vi "Init.vi"(11 "Online?":bool) -> (0 "Fehler out":T1, 1 "SPS-Event":refnum<user-event>, 2 "Version":string, 3 "Cluster out":T2={"Initialisierung"={"Online?"=FALSE, "Grundpfad"=path "", "Kamera Oben"="", "IP-Adresse Flüssiglinse"="", "Flüssiglinse"=refnum, "Kamera Unten"="", "IP-Adresse SPS"="", "SPS-Verbindung"={"TCP Connection Ref"=refnum, "IP address"="", "timeout ms"=5000, "Connected?"=FALSE, "PLC Type"=enum."S7 1200", "Rack S7 400"=0, "Slot S7 400"=0, "PDU Size"=0, "connection semaphore"=refnum}, "IP-Adresse Lichtgitter"="", "Lichtgitter"=refnum, "Skalierungsfaktor"=0.0, "Bilder Oben"=[], "Bild Unten"=refnum, "Bild Ausschnitt Unten"=refnum}, "Einstellungen"={"Gesamtablauf gestartet"=FALSE, "i. O. Bilder speichern"=FALSE, "Bildspeicherung Offline"=FALSE, "Ausgewähltes Offline-Datum"="", "Ausgewähltes Offline-Teil"="", "Speicherpfad Bilder"=path ""}, "Artikeldaten"={"Artikelnummer"="", "Fertigungsauftrag"="", "Muster ISO"=refnum, "Belichtungszeit Referenzmarken"=0.0, "Fokus Referenzmarken"=0.0, "Belichtungszeit ISO"=0.0, "Fokus ISO"=0.0, "Belichtungszeit Unten"=0.0, "Kontaktanzahl"=0, "Aktueller Kontakt"=0, "Kontaktposition"={"x"=0.0, "y"=0.0}, "Winkel ISO"=0.0, "ISO-Muster nicht vorhanden"=FALSE}, "Werte Kamera Oben"={"Koordinatensystem"={"Punkt x-Achse"={"X"=0.0, "Y"=0.0}, "Ursprung"={"X"=0.0, "Y"=0.0}, "Punkt y-Achse"={"X"=0.0, "Y"=0.0}}, "Position Kontakt"={"x"=0.0, "y"=0.0}, "Winkel Kontakt"=0.0}, "Werte Kamera Unten"={"Prüfung Unten n. i. O."=FALSE}, "Werte Lichtgitter"={"Messwerte Referenzmarken"=[], "Mittelpunkt Referenzmarken"={"x"=0.0, "y"=0.0}, "Messwerte Kontakt"=[], "Offset"={"x"=0.0, "y"=0.0}}, "Rückmeldungen"={"Koordinaten ermittelt"=FALSE, "Vermessung Lichtgitter fertig"=FALSE, "Nachkontrolle Kamera Unten fertig"=FALSE}, "Fehler"={"Referenzen nicht gefunden"=FALSE, "Kontakt nicht gefunden"=FALSE, "Referenzen nicht in Lichtgitter"=FALSE, "Kontakt zu groß"=FALSE, "Kontakt zu klein"=FALSE}, "Statistik"={"Statistiken"=[]}, "Timer"={"Timer Start Position"=0, "Timer Start Lichtgitter"=0, "Timer Start Kamera Unten"=0}})   [LabVIEW 2024]
doc: "Verbindet alle Geräte und initialisiert Grundvariablen"
uses:
  Cluster.ctl
  Kontaktmontagemodul.exe/1abvi3w/vi.lib/userDefined/High Color/IMAQdx.ctl
  Kontaktmontagemodul.exe/1abvi3w/vi.lib/DATA AHEAD/SP7/typedefs/S7 Connection.ctl
  Kontaktmontagemodul.exe/1abvi3w/vi.lib/DATA AHEAD/SP7/typedefs/PLC Type.ctl
  Kontaktmontagemodul.exe/1abvi3w/vi.lib/vision/Image Controls.llb/IMAQ Image.ctl
  Koordinatensystem.ctl
  Statistik.ctl
  Cluster_Fehler_Initialisierung.ctl
  Zustand.ctl
  Globale Variablen.vi
  Kontaktmontagemodul.exe/1abvi3w/vi.lib/DATA AHEAD/SP7/SP7.lvlib
  Kontaktmontagemodul.exe/1abvi3w/vi.lib/vision/driver/NI_Vision_Acquisition_Software.lvlib
  Kontaktmontagemodul.exe/1abvi3w/vi.lib/Utility/config.llb/NI_LVConfig.lvlib
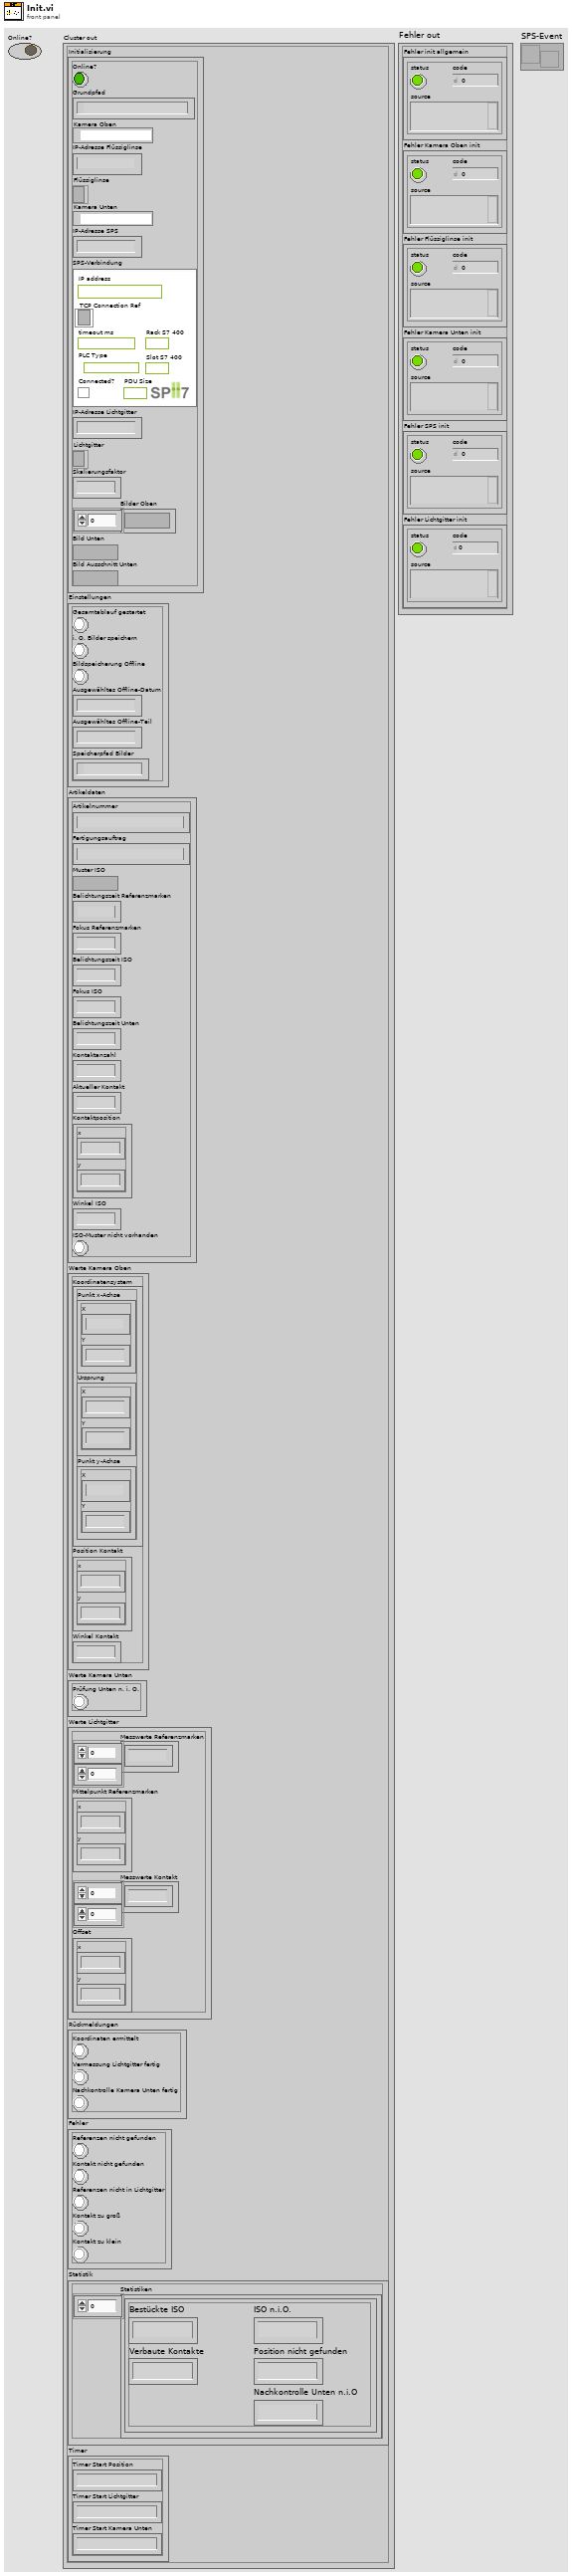
[diagram p1: front panel]
types:
  T1 = typedef "Cluster_Fehler_Initialisierung.ctl" = cluster{"Fehler init allgemein":errorcluster, "Fehler Kamera Oben init":errorcluster, "Fehler Flüssiglinse init":errorcluster, "Fehler Kamera Unten init":errorcluster, "Fehler SPS init":errorcluster, "Fehler Lichtgitter init":errorcluster}
  T2 = typedef "Cluster.ctl" = cluster{"Initialisierung":cluster{"Online?":bool, "Grundpfad":path, "Kamera Oben":T3, "IP-Adresse Flüssiglinse":string, "Flüssiglinse":refnum<k5>, "Kamera Unten":T3, "IP-Adresse SPS":string, "SPS-Verbindung":T4, "IP-Adresse Lichtgitter":string, "Lichtgitter":refnum<k5>, "Skalierungsfaktor":dbl, "Bilder Oben":T7[], "Bild Unten":T7, "Bild Ausschnitt Unten":T7}, "Einstellungen":cluster{"Gesamtablauf gestartet":bool, "i. O. Bilder speichern":bool, "Bildspeicherung Offline":bool, "Ausgewähltes Offline-Datum":string, "Ausgewähltes Offline-Teil":string, "Speicherpfad Bilder":path}, "Artikeldaten":cluster{"Artikelnummer":string, "Fertigungsauftrag":string, "Muster ISO":T7, "Belichtungszeit Referenzmarken":dbl, "Fokus Referenzmarken":dbl, "Belichtungszeit ISO":dbl, "Fokus ISO":dbl, "Belichtungszeit Unten":dbl, "Kontaktanzahl":u32, "Aktueller Kontakt":i16, "Kontaktposition":cluster{"x":sgl, "y":sgl}, "Winkel ISO":sgl, "ISO-Muster nicht vorhanden":bool}, "Werte Kamera Oben":cluster{"Koordinatensystem":T8, "Position Kontakt":cluster{"x":dbl, "y":dbl}, "Winkel Kontakt":dbl}, "Werte Kamera Unten":cluster{"Prüfung Unten n. i. O.":bool}, "Werte Lichtgitter":cluster{"Messwerte Referenzmarken":dbl[][], "Mittelpunkt Referenzmarken":cluster{"x":dbl, "y":dbl}, "Messwerte Kontakt":dbl[][], "Offset":cluster{"x":dbl, "y":dbl}}, "Rückmeldungen":cluster{"Koordinaten ermittelt":bool, "Vermessung Lichtgitter fertig":bool, "Nachkontrolle Kamera Unten fertig":bool}, "Fehler":cluster{"Referenzen nicht gefunden":bool, "Kontakt nicht gefunden":bool, "Referenzen nicht in Lichtgitter":bool, "Kontakt zu groß":bool, "Kontakt zu klein":bool}, "Statistik":cluster{"Statistiken":T9[]}, "Timer":cluster{"Timer Start Position":u32, "Timer Start Lichtgitter":u32, "Timer Start Kamera Unten":u32}}
  T3 = typedef "IMAQdx.ctl" = refnum<k21>
  T4 = typedef "SP7.lvlib/S7 Connection.ctl" = cluster{"TCP Connection Ref":refnum<k5>, "IP address":string, "timeout ms":i32, "Connected?":bool, "PLC Type":T5, "Rack S7 400":u8, "Slot S7 400":u8, "PDU Size":u16, "connection semaphore":T6}
  T5 = typedef "SP7.lvlib/PLC Type.ctl" = enum16{"S7 200", "S7 300/400", "S7 1200", "S7 1500", "LOGO!8"}
  T6 = typedef "Semaphore RefNum" = refnum<k1>
  T7 = typedef "IMAQ Image.ctl" = refnum<image>
  T8 = typedef "Koordinatensystem.ctl" = cluster{"Punkt x-Achse":cluster{"X":sgl, "Y":sgl}, "Ursprung":cluster{"X":sgl, "Y":sgl}, "Punkt y-Achse":cluster{"X":sgl, "Y":sgl}}
  T9 = typedef "Statistik.ctl" = cluster{"Bestückte ISO":u32, "Verbaute Kontakte":u32, "ISO n.i.O.":u32, "Nachkontrolle Unten n.i.O":u32, "Position nicht gefunden":u32}
  T10 = typedef "Zustand.ctl" = enum16{"Warten auf Event", "Artikeldaten laden", "Init Prüfung Oben", "Bildaufnahme Oben", "Auswertung Oben", "Bilder Oben speichern", "Init Vermessung Lichtgitter", "Messwertaufnahme Lichtgitter", "Auswertung Lichtgitter", "Init Prüfung Unten", "Bildaufnahme Unten", "Auswertung Unten", "Bild Unten speichern", "Update Statistik", "Fehler quittieren"}
  T11 = typedef "NI_LVConfig.lvlib/Config Data RefNum.ctl" = refnum<k1>
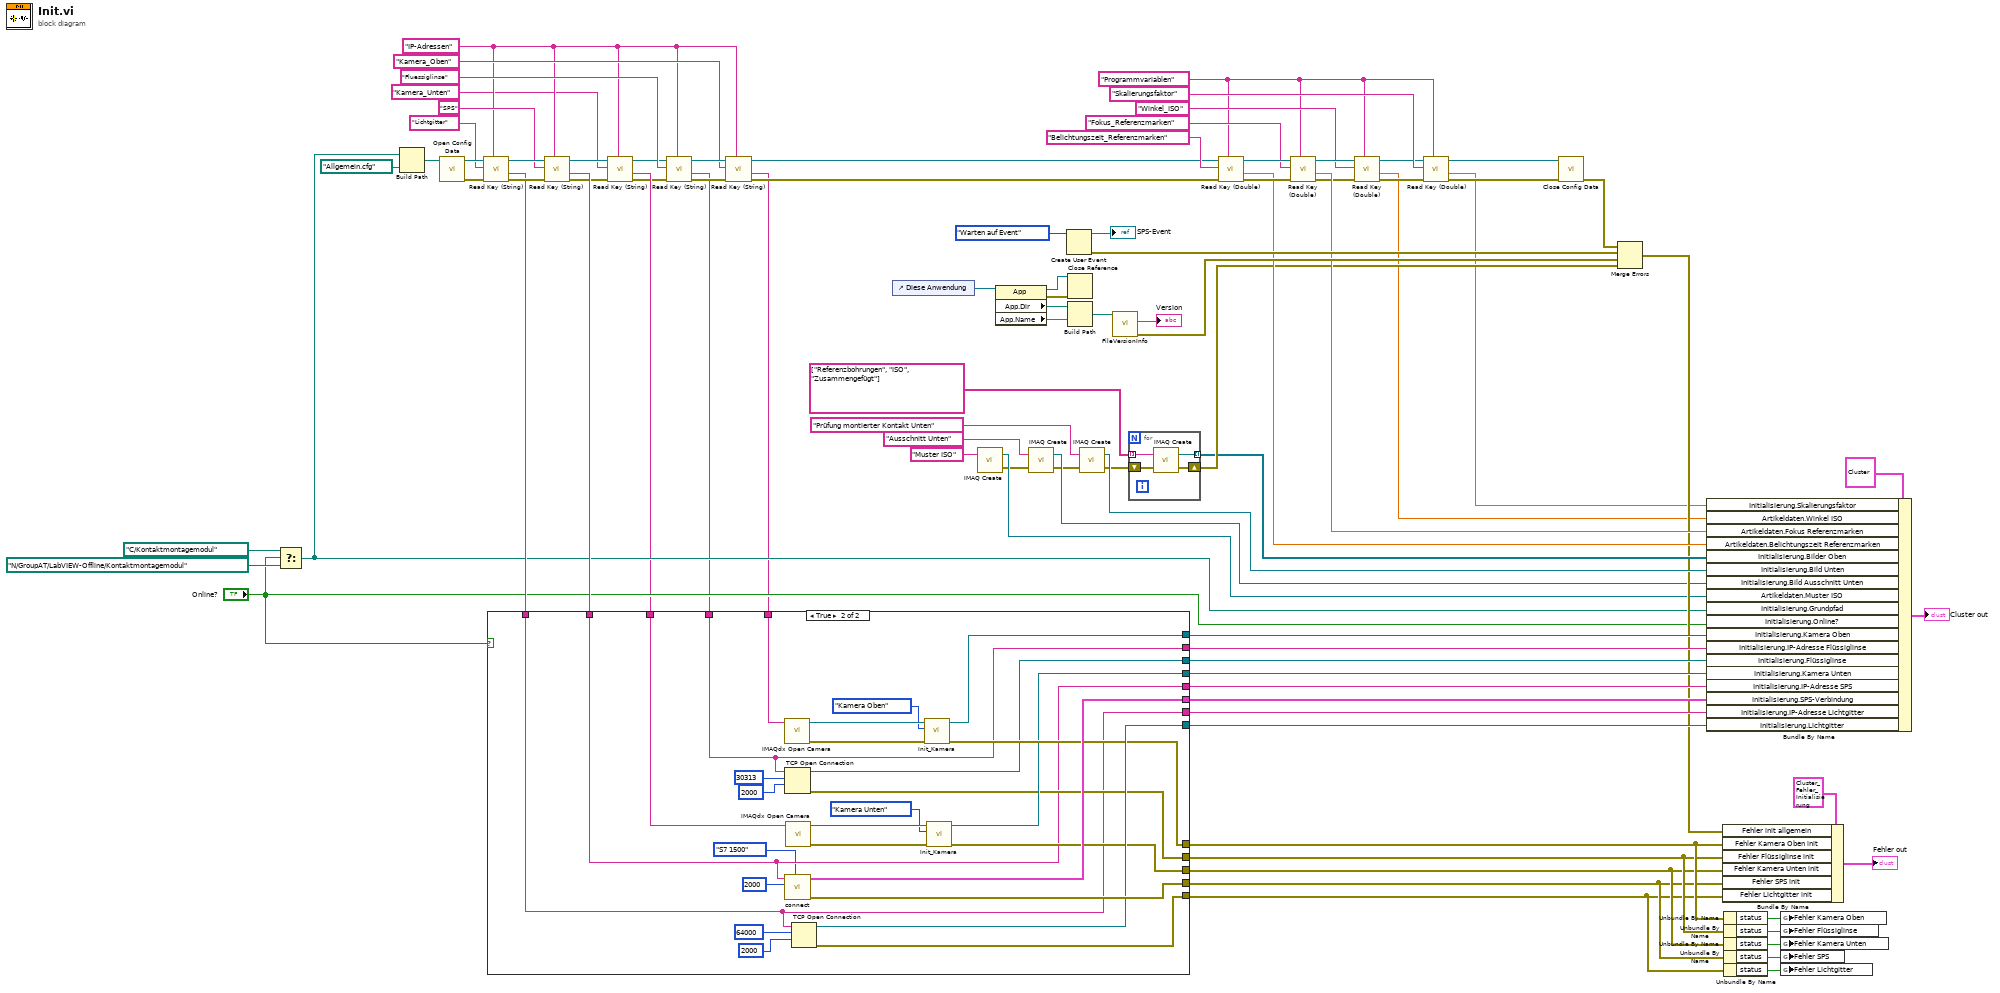
[diagram p0: block diagram]
diagram:
  w21 = "IP-Adressen" ("section")
  w3 = "Programmvariablen" ("section")
  n1 = Select(t=path "C:/Kontaktmontagemodul", s="Online?", f=path "N:/GroupAT/LabVIEW-Offline/Kontaktmontagemodul") -> (s? t:f=w33:path)
  n2 = Build Path(base path=w33, name or relative path=path "Allgemein.cfg") -> (appended path=w67:path)
  n3 = call "Open Config Data.vi"("configuration file path"=w67) -> ("error out"=w52:errorcluster, "refnum"=w53:T11)  [unwired: 8 in, 1 out]
  n4 = call "Read Key (String).vi"("section"=w21, "error in (no error)"=w52, "key"="Lichtgitter", "refnum"=w53) -> ("error out"=w50:errorcluster, "value"=w45:string, "refnum out"=w51:T11)  [unwired: 4 in, 1 out]
  n5 = call "Read Key (String).vi"("section"=w21, "error in (no error)"=w50, "key"="SPS", "refnum"=w51) -> ("error out"=w22:errorcluster, "value"=w46:string, "refnum out"=w26:T11)  [unwired: 4 in, 1 out]
  n6 = call "Read Key (String).vi"("section"=w21, "error in (no error)"=w22, "key"="Kamera_Unten", "refnum"=w26) -> ("error out"=w23:errorcluster, "value"=w24:string, "refnum out"=w25:T11)  [unwired: 4 in, 1 out]
  n7 = call "Read Key (String).vi"("section"=w21, "error in (no error)"=w23, "key"="Fluessiglinse", "refnum"=w25) -> ("error out"=w32:errorcluster, "value"=w19:string, "refnum out"=w31:T11)  [unwired: 4 in, 1 out]
  n8 = call "Read Key (String).vi"("section"=w21, "error in (no error)"=w32, "key"="Kamera_Oben", "refnum"=w31) -> ("error out"=w29:errorcluster, "value"=w28:string, "refnum out"=w30:T11)  [unwired: 4 in, 1 out]
  n9 = case shown="True" "Online?" {
    tunnel: [_ w120] -> w36
    tunnel: [_ w112] -> w44
    tunnel: [_ w119] -> w35
    tunnel: [_ w107] -> w37
    tunnel: [_ w110] -> w85
    tunnel: [_ w106] -> w84
    tunnel: [_ w118] -> w83
    tunnel: [_ w117] -> w82
    tunnel: [_ w98] -> w74
    tunnel: [_ w97] -> w75
    tunnel: [_ w102] -> w73
    tunnel: [_ w99] -> w72
    tunnel: [_ w101] -> w38
    tunnel: w19 -> [_ w99]
    tunnel: w46 -> [_ w98]
    tunnel: w45 -> [_ w97]
    tunnel: w28 -> [_ w96]
    tunnel: w24 -> [_ w95]
    frame False {
    }
    frame True {
      n10 = call "IMAQdx Open Camera.vi"("Session In"=w96) -> ("error out"=w113:errorcluster, "Session Out"=w111:T3)  [unwired: 9 in]
      n11 = TCP Open Connection(address=w99, remote port or service name=u16 30313 ("Netzwerk-Port oder -Dienst"), timeout ms (60000)=2000) -> (connection ID=w102:refnum<k5>, error out=w101:errorcluster)  [unwired: 2 in]
      n12 = call "connect.vi"("PLC Type"=PLC_Type."S7 1500", "timeout [ms]"=2000, "IP address"=w98) -> ("error out"=w120:errorcluster, "S7 Connection out"=w118:T4)  [unwired: 7 in]
      n13 = call "IMAQdx Open Camera.vi"("Session In"=w95) -> ("error out"=w109:errorcluster, "Session Out"=w108:T3)  [unwired: 9 in]
      n14 = TCP Open Connection(address=w97, remote port or service name=u16 64000, timeout ms (60000)=2000) -> (connection ID=w117:refnum<k5>, error out=w119:errorcluster)  [unwired: 2 in]
      n15 = call "Init_Kamera.vi"("Fehler in"=w113, "Kamera"=enum16{"Kamera Oben", "Kamera Unten"}."Kamera Oben", "Kamera in"=w111) -> ("Fehler out"=w112:errorcluster, "Kamera out"=w110:T3)  [unwired: 7 in]
      n16 = call "Init_Kamera.vi"("Fehler in"=w109, "Kamera"=enum16{"Kamera Oben", "Kamera Unten"}."Kamera Unten", "Kamera in"=w108) -> ("Fehler out"=w107:errorcluster, "Kamera out"=w106:T3)  [unwired: 7 in]
    }
  }
  n17 = control-ref of="Diese Anwendung"() -> (w93:refnum<vi>)
  n18 = call "IMAQ Create"("Image Name"="Muster ISO") -> ("New Image"=w7:T7, "error out"=w6:errorcluster)  [unwired: 4 in]
  n19 = property class="App"(reference=w93) -> (reference out=w89:refnum<vi>, error out=w90:errorcluster, "App.Dir"=w91:path, "App.Name"=w92:string)  [unwired: 1 in]
  n20 = call "IMAQ Create"("Image Name"="Ausschnitt Unten", "error in (no error)"=w6) -> ("New Image"=w14:T7, "error out"=w5:errorcluster)  [unwired: 3 in]
  n21 = Create User Event(user event datatype=Zustand."Warten auf Event" ("Enum")) -> (user event=→"SPS-Event":refnum<user-event>, error out=w70:errorcluster)  [unwired: 1 in]
  n22 = Close Reference(reference=w89, error in (no error)=w90) -> ()  [unwired: 1 out]
  n23 = Build Path(base path=w91, name or relative path=w92) -> (appended path=w88:path)
  n24 = call "IMAQ Create"("Image Name"="Prüfung montierter Kontakt Unten", "error in (no error)"=w5) -> ("New Image"=w77:T7, "error out"=w4:errorcluster)  [unwired: 3 in]
  n25 = call "FileVersionInfo.vi"("Application Path in"=w88) -> ("error out"=w79:errorcluster, "File Version Info"=→"Version":string)  [unwired: 7 in, 2 out]
  n26 = for {
    shift-right: [w124] -> w58
    shift-left: w4 -> [w123]
    tunnel: string[] ["Referenzbohrungen", "ISO", "Zusammengefügt"] -> [w122] mode=indexing
    tunnel: [w121] -> w57 mode=indexing
    n27 = call "IMAQ Create"("Image Name"=w122, "error in (no error)"=w123) -> ("New Image"=w121:T7, "error out"=w124:errorcluster)  [unwired: 3 in]
  }
  n28 = call "Read Key (Double).vi"("section"=w3, "error in (no error)"=w29, "key"="Belichtungszeit_Referenzmarken", "refnum"=w30) -> ("error out"=w63:errorcluster, "value"=w61:dbl, "refnum out"=w64:T11)  [unwired: 4 in, 1 out]
  n29 = call "Read Key (Double).vi"("section"=w3, "error in (no error)"=w63, "key"="Fokus_Referenzmarken", "refnum"=w64) -> ("error out"=w11:errorcluster, "value"=w60:dbl, "refnum out"=w13:T11)  [unwired: 4 in, 1 out]
  n30 = call "Read Key (Double).vi"("section"=w3, "error in (no error)"=w11, "key"="Winkel_ISO", "refnum"=w13) -> ("error out"=w10:errorcluster, "value"=w8:dbl, "refnum out"=w12:T11)  [unwired: 4 in, 1 out]
  n31 = call "Read Key (Double).vi"("section"=w3, "error in (no error)"=w10, "key"="Skalierungsfaktor" ("section"), "refnum"=w12) -> ("error out"=w17:errorcluster, "value"=w2:dbl, "refnum out"=w18:T11)  [unwired: 4 in, 1 out]
  n32 = call "Close Config Data.vi"("error in (no error)"=w17, "refnum"=w18) -> ("error out"=w66:errorcluster)  [unwired: 8 in, 1 out]
  n33 = Merge Errors(w66, w70, w79, w58) -> (w56:errorcluster)
  n34 = Bundle By Name(cluster=T2 {"Initialisierung"={"Online?"=FALSE, "Grundpfad"=path "N:/GroupAT/LabVIEW-Offline/Kontaktmontagemodul", "Kamera Oben"="", "IP-Adresse Flüssiglinse"="", "Flüssiglinse"=refnum, "Kamera Unten"="", "IP-Adresse SPS"="", "SPS-Verbindung"={"TCP Connection Ref"=refnum, "IP address"="", "timeout ms"=0, "Connected?"=FALSE, "PLC Type"=enum."S7 200", "Rack S7 400"=0, "Slot S7 400"=0, "PDU Size"=0, "connection semaphore"=refnum}, "IP-Adresse Lichtgitter"="", "Lichtgitter"=refnum, "Skalierungsfaktor"=0.0, "Bilder Oben"=["remote image 00000000108EE02C", "remote image 00000000108EE12C", "remote image 00000000108EE82C"], "Bild Unten"="remote image 00000000108EE1AC", "Bild Ausschnitt Unten"=refnum}, "Einstellungen"={"Gesamtablauf gestartet"=FALSE, "i. O. Bilder speichern"=FALSE, "Bildspeicherung Offline"=FALSE, "Ausgewähltes Offline-Datum"="12.07.24", "Ausgewähltes Offline-Teil"="0", "Speicherpfad Bilder"=path "N:/GroupAT/LabVIEW-Offline/Kontaktmontagemodul/Artikelnummern/Test/Bilder/23.08.24/2"}, "Artikeldaten"={"Artikelnummer"="", "Fertigungsauftrag"="", "Muster ISO"=refnum, "Belichtungszeit Referenzmarken"=1000.0, "Fokus Referenzmarken"=-2.0, "Belichtungszeit ISO"=0.0, "Fokus ISO"=0.0, "Belichtungszeit Unten"=0.0, "Kontaktanzahl"=0, "Aktueller Kontakt"=1, "Kontaktposition"={"x"=0.0, "y"=0.0}, "Winkel ISO"=0.0, "ISO-Muster nicht vorhanden"=FALSE}, "Werte Kamera Oben"={"Koordinatensystem"={"Punkt x-Achse"={"X"=0.0, "Y"=0.0}, "Ursprung"={"X"=0.0, "Y"=0.0}, "Punkt y-Achse"={"X"=0.0, "Y"=0.0}}, "Position Kontakt"={"x"=0.0, "y"=0.0}, "Winkel Kontakt"=0.0}, "Werte Kamera Unten"={"Prüfung Unten n. i. O."=FALSE}, "Werte Lichtgitter"={"Messwerte Referenzmarken"=[], "Mittelpunkt Referenzmarken"={"x"=0.0, "y"=0.0}, "Messwerte Kontakt"=[], "Offset"={"x"=0.0, "y"=0.0}}, "Rückmeldungen"={"Koordinaten ermittelt"=FALSE, "Vermessung Lichtgitter fertig"=FALSE, "Nachkontrolle Kamera Unten fertig"=FALSE}, "Fehler"={"Referenzen nicht gefunden"=FALSE, "Kontakt nicht gefunden"=FALSE, "Referenzen nicht in Lichtgitter"=FALSE, "Kontakt zu groß"=FALSE, "Kontakt zu klein"=FALSE}, "Statistik"={"Statistiken"=[]}, "Timer"={"Timer Start Position"=0, "Timer Start Lichtgitter"=0, "Timer Start Kamera Unten"=0}} ("Cluster out"), "Initialisierung.Skalierungsfaktor"=w2, "Artikeldaten.Winkel ISO"=w8, "Artikeldaten.Fokus Referenzmarken"=w60, "Artikeldaten.Belichtungszeit Referenzmarken"=w61, "Initialisierung.Bilder Oben"=w57, "Initialisierung.Bild Unten"=w77, "Initialisierung.Bild Ausschnitt Unten"=w14, "Artikeldaten.Muster ISO"=w7, "Initialisierung.Grundpfad"=w33, "Initialisierung.Online?"="Online?", "Initialisierung.Kamera Oben"=w85, "Initialisierung.IP-Adresse Flüssiglinse"=w72, "Initialisierung.Flüssiglinse"=w73, "Initialisierung.Kamera Unten"=w84, "Initialisierung.IP-Adresse SPS"=w74, "Initialisierung.SPS-Verbindung"=w83, "Initialisierung.IP-Adresse Lichtgitter"=w75, "Initialisierung.Lichtgitter"=w82) -> (→"Cluster out":T2)
  n35 = Bundle By Name(cluster=T1 {"Fehler init allgemein"={"status"=FALSE, "code"=0, "source"=""}, "Fehler Kamera Oben init"={"status"=FALSE, "code"=0, "source"=""}, "Fehler Flüssiglinse init"={"status"=FALSE, "code"=0, "source"=""}, "Fehler Kamera Unten init"={"status"=FALSE, "code"=0, "source"=""}, "Fehler SPS init"={"status"=FALSE, "code"=0, "source"=""}, "Fehler Lichtgitter init"={"status"=FALSE, "code"=0, "source"=""}} ("Cluster"), "Fehler init allgemein"=w56, "Fehler Kamera Oben init"=w44, "Fehler Flüssiglinse init"=w38, "Fehler Kamera Unten init"=w37, "Fehler SPS init"=w36, "Fehler Lichtgitter init"=w35) -> (→"Fehler out":T1)
  n36 = Unbundle By Name(w44) -> ("status"=w43:bool)
  n37 = Unbundle By Name(w38) -> ("status"=w42:bool)
  n38 = Unbundle By Name(w37) -> ("status"=w41:bool)
  n39 = Unbundle By Name(w36) -> ("status"=w40:bool)
  n40 = Unbundle By Name(w35) -> ("status"=w39:bool)
  n41 = global write "Globale Variablen.vi" "Fehler Kamera Oben"(w43) -> ()
  n42 = global write "Globale Variablen.vi" "Fehler Flüssiglinse"(w42) -> ()
  n43 = global write "Globale Variablen.vi" "Fehler Kamera Unten"(w41) -> ()
  n44 = global write "Globale Variablen.vi" "Fehler SPS"(w40) -> ()
  n45 = global write "Globale Variablen.vi" "Fehler Lichtgitter"(w39) -> ()
